vi "Get Result.vi"(6 "timeout (ms)":i32=5000, 8 "error in":errorcluster, 11 "gRPC ID":T1) -> (0 "error out":errorcluster, 2 "result":i32, 3 "gRPC ID out":T1)   [LabVIEW 2021, in "CIFTemplateWrapper.lvlib"]
uses:
  CIFTemplateWrapper.lvlib
  <vilib>/gRPC/LabVIEW gRPC Library/Shared/grpcId.ctl
  CIFTemplatePlugin_client/CIFTemplatePlugin_client.lvlib
  <vilib>/gRPC/LabVIEW gRPC Library/grpc-lvsupport-release.lvlib
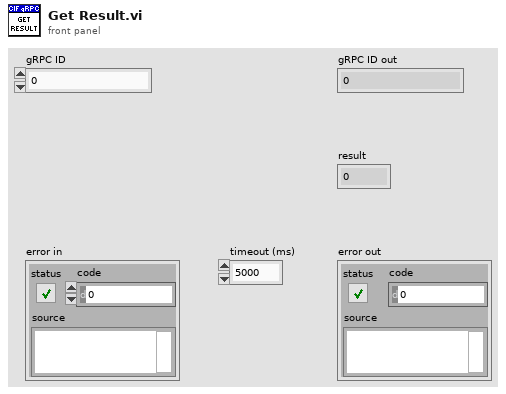
[diagram p1: front panel]
types:
  T1 = typedef "grpc-lvsupport-release.lvlib/grpcId.ctl" = u64
  T2 = typedef "CIFTemplatePlugin_client.lvlib/cif_templateplugin_Result.ctl" = cluster{"result":i32}
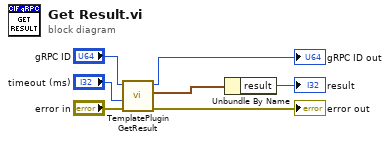
[diagram p0: block diagram]
diagram:
  n1 = call "TemplatePlugin GetResult.vi"("error in"="error in", "timeout (ms)"="timeout (ms)", "gRPC ID"="gRPC ID") -> ("error out"=→"error out":errorcluster, "Response Data"=w1:T2, "gRPC ID out"=→"gRPC ID out":T1)  [unwired: 6 in]
  n2 = Unbundle By Name(w1) -> ("result"=→"result":i32)
